vi "practice.vi"() -> ()   [LabVIEW 2020]
uses:
  7409fd4a-f124-4f99-9fbe-ba52ef24ff4a.vi
  <vilib>/Comparison/Less/Less Functor/Less Functor.lvclass
panel:
  out "Array 2":i32[](array[numeric])
  in  "Array":dbl[](array[numeric])
  out "sum":dbl
  out "Numeric 2":dbl
  out "Numeric":dbl
  out "Boolean 7":bool
  out "Boolean 6":bool
  out "Boolean 5":bool
  out "Boolean 4":bool
  out "Boolean 3":bool
  out "Boolean 2":bool
  out "Boolean":bool
  out "sorted array":i32[](array[numeric])
  out "Ascending":i32[](array[numeric])
  out "Tables":i32[](array[numeric])
  out "ODD":dbl[](array[numeric])
  out "EVEN":dbl[](array[numeric])
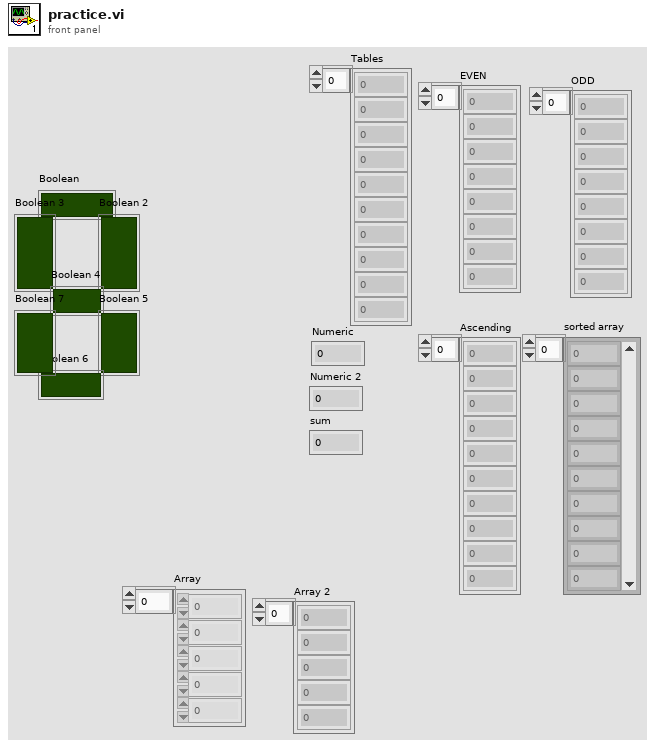
[diagram p1: front panel]
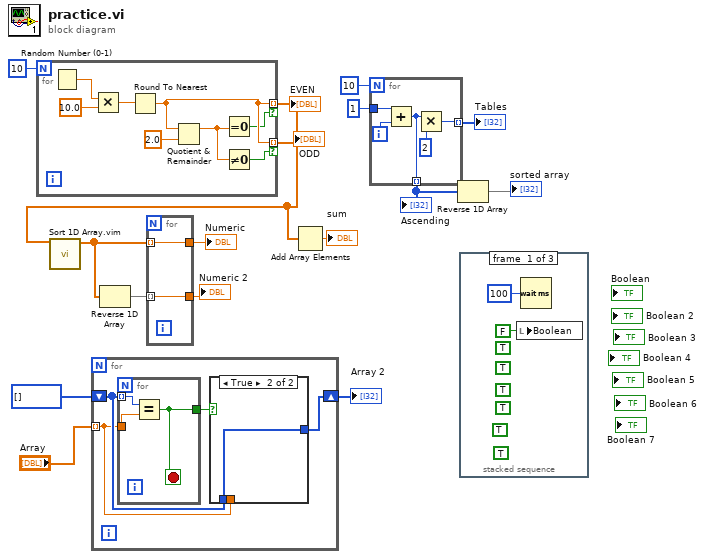
[diagram p0: block diagram]
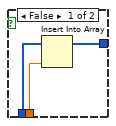
[diagram p2: hidden frame]
diagram:
  n1 = for {
    N: 10 -> [_]
    tunnel: [w21] -> w5 mode=indexing if=w19
    tunnel: [w21] -> w15 mode=indexing if=w18
    n2 = Random Number (0-1)() -> (number: 0 to 1=w24:dbl)
    n3 = Multiply(x=w24, y=10.0) -> (x*y=w22:dbl)
    n4 = Round To Nearest(number=w22) -> (nearest integer value=w21:dbl)
    n5 = Quotient & Remainder(x=w21, y=2.0) -> (x-y*floor(x/y)=w17:dbl)  [unwired: 1 out]
    n6 = Equal To 0?(x=w17) -> (x = 0?=w19:bool)
    n7 = Not Equal To 0?(x=w17) -> (x != 0?=w18:bool)
  }
  "EVEN" <- w5
  "ODD" <- w15
  n8 = call "Sort 1D Array.vim"("unsorted array"=w5) -> ("sorted array"=w9:dbl[])  [unwired: 10 in]
  n9 = for {
    tunnel: "Array" -> [w26] mode=indexing
    shift-right: [w25] -> w1
    shift-left: i32[] [] -> [w27]
    n10 = for {
      tunnel: w26 -> [w34]
      tunnel: w27 -> [w35] mode=indexing
      tunnel: [w33] -> w28
      stop <- w33 stop-if-true
      n11 = Equal?(x=w35, y=w34) -> (x = y?=w33:bool)
    }
    n12 = case shown="True" w28 {
      tunnel: w27 -> [w31 w32]
      tunnel: w26 -> [w30 _]
      tunnel: [w29 w32] -> w25
      frame False {
        n13 = Insert Into Array(array=w31, new element=w30) -> (w29:i32[])  [unwired: 1 in]
      }
      frame True {
      }
    }
  }
  "Array 2" <- w1
  n14 = Reverse 1D Array(array=w9) -> (reversed array=w8:dbl[])
  n15 = for {
    tunnel: w9 -> [w37] mode=indexing
    tunnel: w8 -> [w36] mode=indexing
    tunnel: [w37] -> w7
    tunnel: [w36] -> w6
  }
  "Numeric" <- w7
  "Numeric 2" <- w6
  n16 = Add Array Elements(numeric array=w5) -> (sum=→"sum":dbl)
  n17 = for {
    N: 10 -> [_]
    tunnel: 1 -> [w42]
    tunnel: [w39] -> w12 mode=indexing
    tunnel: [w38] -> w11 mode=indexing
    i -> [w41]
    n18 = Add(x=w42, y=w41) -> (x+y=w38:i32)
    n19 = Multiply(x=w38, y=2) -> (x*y=w39:i32)
  }
  "Tables" <- w12
  "Ascending" <- w11
  n20 = Reverse 1D Array(array=w11) -> (reversed array=→"sorted array":i32[])
  n21 = stacked-sequence {
    frame #0 {
      (unwired) TRUE
      (unwired) TRUE
      (unwired) TRUE
      (unwired) TRUE
      (unwired) TRUE
      (unwired) TRUE
      n22 = local write "Boolean"(FALSE) -> ()
      n23 = Wait (ms)(milliseconds to wait=u32 100) -> ()  [unwired: 1 out]
    }
    frame #1 {
    }
    frame #2 {
    }
  }
